vi "LV to ITX  Retrieve.vi"(0 "File or Folder Path":path, 1 "Data Type":T1=enum."TDMS", 2 "DAT header length":i32=11, 5 "offset":i32, 7 "length":i32=1, 9 "index":T2={"A"=10, "B"=6, "C"=14, "D"=1, "E"=2, "N1"=3, "N2"=2, "N3"=0, "N4"=0}, 11 "error in (no error)":errorcluster) -> (4 "A vs B":cluster{dbl[], dbl[]}[](graph), 6 "C vs D":cluster{dbl[], dbl[]}[](graph), 8 "E":dbl[][](graph), 10 "N":cluster{"N1":dbl, "N2":dbl, "N3":dbl, "N4":dbl}={"N1"=0.0624995231628418, "N2"=0.0624995231628418, "N3"=0.0624995231628418, "N4"=0.0624995231628418} {"N4" format="%#_6p"; "N3" format="%#_6p"; "N2" format="%#_6p"; "N1" format="%#_6p"}, 14 "Comments":string)   [LabVIEW 2020, in "LVtoITX.lvclass"]
uses:
  <userlib>/LevyLab/LV to ITX/LVtoITX.lvclass
  <userlib>/LevyLab/LV-Data/LV-Data.ITX/LV-Data.ITX.lvclass
  <userlib>/LevyLab/LV-Data/LV-Data.TDMS/LV-Data.TDMS.lvclass
  <userlib>/LevyLab/Graph Utilities/graph_utilities.lvclass
  <vilib>/Utility/miscctls.llb/LVOffsetAndMultiplierTypeDef.ctl
  <userlib>/LevyLab/LV-Data/LV-Data.ITX/Typedefs/Retrieve Data Type.ctl
panel:
  in  "D  is time?":bool
  in  "B is time?":bool
  out "time":string[][](table)
  in  "Use Folder Index File?":bool
  in  "Generate Folder Index File?":bool
  in  "Ez name":string="Ez name"
  in  "Ey name":string="Ey name"
  in  "Ex name":string="Ex name"
  in  "C y name":string="C y name"
  in  "D x name":string="D x name"
  in  "A y name":string="A y name"
  in  "B x name":string="B x name"
  out "Index, Wavenames":string[][](table)=[["0", "Time"], ["1", "Vsg"], ["2", "X1"], ["3", "Y1"], ["4", "X2"], ["5", "Y2"], ["6", "X3"], ["7", "Y3"], ["8", "X4"], ["9", "Y4"], ["10", "X5"], ["11", "Y5"], ["12", "X6"], ["13", "Y6"], ["14", "X7"], ["15", "Y7"], ["16", "X8"], ["17", "Y8"]]
  in  "recolor traces?":bool
  in  "Ex":T3={"Offset"=0.0, "Multiplier"=1.0}
  in  "Ey":T3={"Offset"=0.0, "Multiplier"=1.0}
  out "Path":path=path "G:/My Drive/ansom/Data/PPMSDAQ/2020/PPMS/SA02821O.20200721/04-Bsweep-Lockin/SA02821O.20200721.000000.tdms"
  out "counter":i32
  out "pattern":string="*.dat"
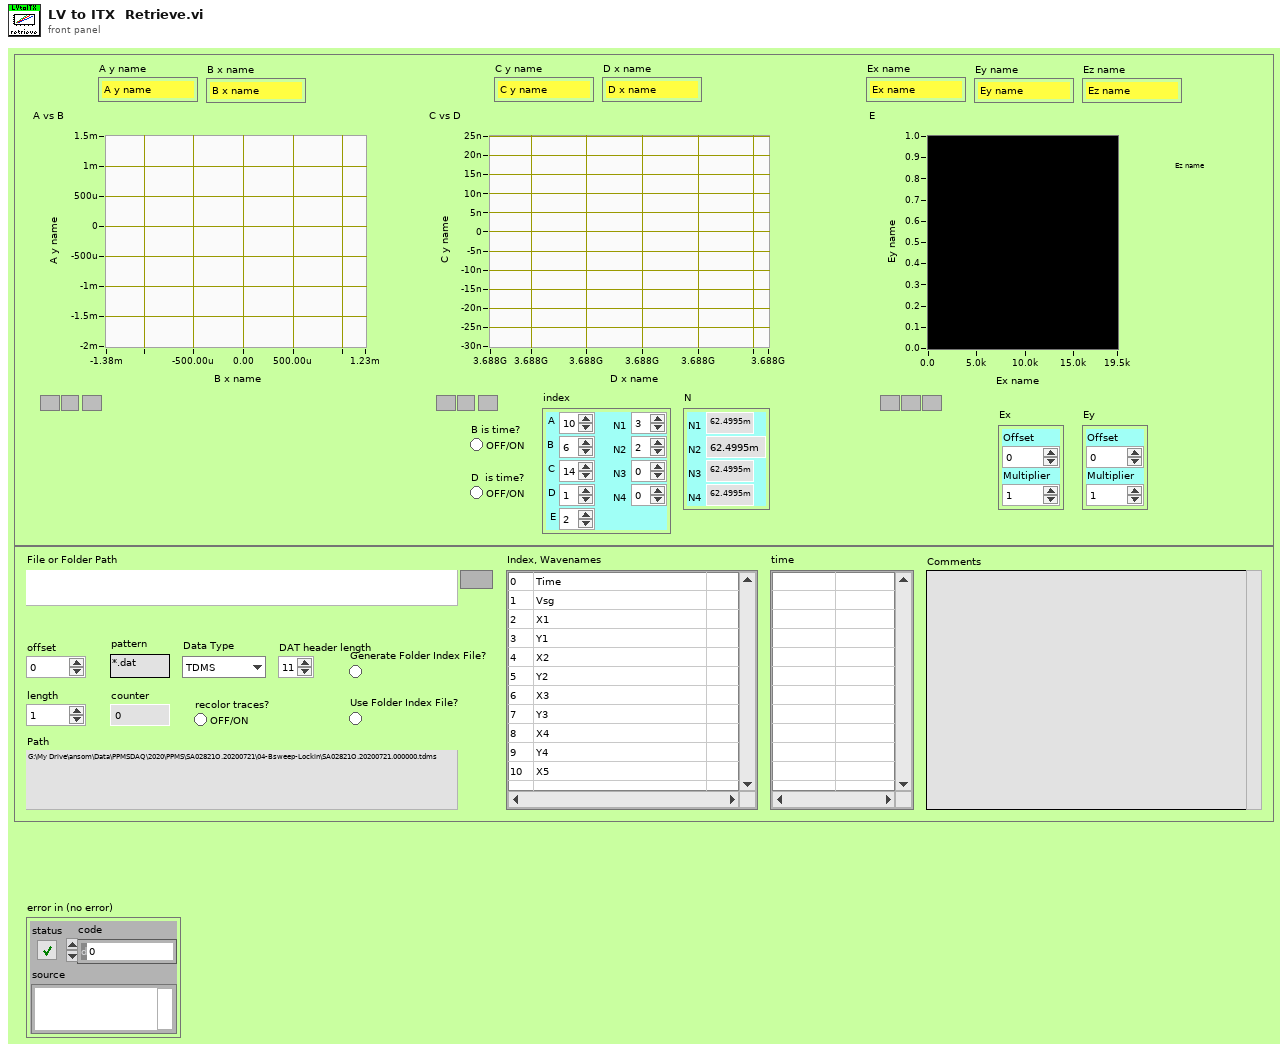
[diagram p1: front panel]
types:
  T1 = typedef "LV-Data.ITX.lvclass/Retrieve Data Type.ctl" = enum16{"ITX", "ITX w/ 2D", "DAT", "TDMS"}
  T2 = cluster{"A":i32, "B":i32, "C":i32, "D":i32, "E":i32, "N1":i32, "N2":i32, "N3":i32, "N4":i32}
  T3 = typedef "LVOffsetAndMultiplierTypeDef.ctl" = cluster{"Offset":dbl, "Multiplier":dbl}
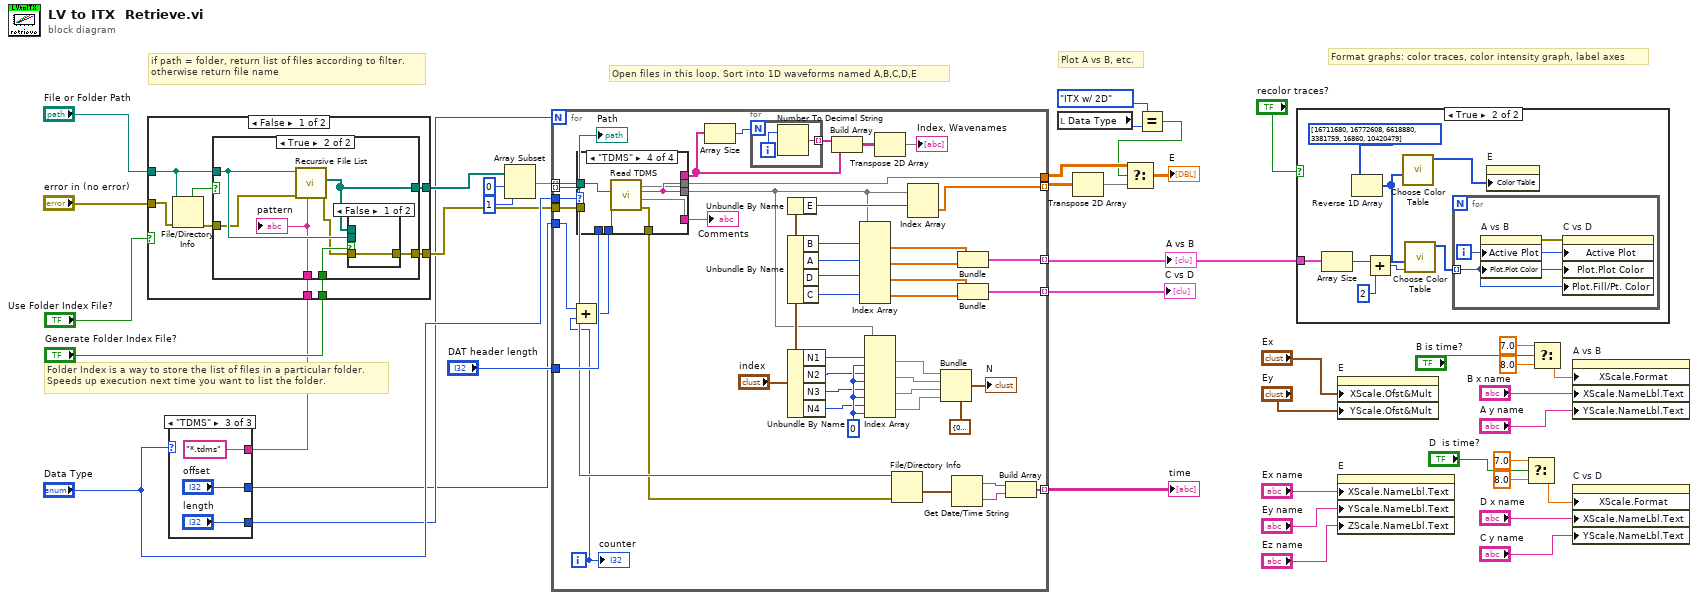
[diagram p0: block diagram]
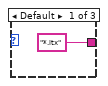
[diagram p2: hidden frame]
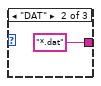
[diagram p3: hidden frame]
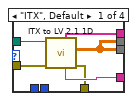
[diagram p5: hidden frame]
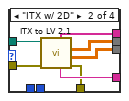
[diagram p6: hidden frame]
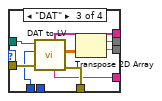
[diagram p7: hidden frame]
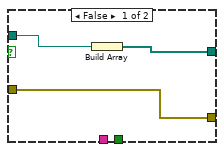
[diagram p8: hidden frame]
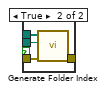
[diagram p9: hidden frame]
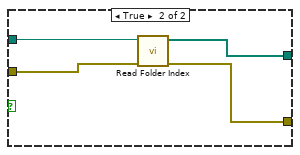
[diagram p10: hidden frame]
diagram:
  # "Plot A vs B, etc."
  # "Format graphs: color traces, color intensity graph, label axes"
  # "Open files in this loop. Sort into 1D waveforms named A,B,C,D,E"
  # "Folder Index is a way to store the list of files in a particular folder.\nSpeeds up execution next time you want to list the folder."
  # "if path = folder, return list of files according to filter.\notherwise return file name"
  n1 = case shown="\"TDMS\"" "Data Type" {
    tunnel: ["*.itx" ("pattern") "*.dat" ("pattern") "*.tdms" ("pattern")] -> w8
    tunnel: [_ _ "length"] -> w2
    tunnel: [_ _ "offset"] -> w1
    frame Default {
    }
    frame "DAT" {
    }
    frame "TDMS" {
    }
  }
  n2 = case shown="False" "Use Folder Index File?" {
    tunnel: [w53 w73] -> w40
    tunnel: "File or Folder Path" -> [w55 w74]
    tunnel: "Generate Folder Index File?" -> [w52 _]
    tunnel: w8 -> [w51 _]
    tunnel: "error in (no error)" -> [w50 w72]
    tunnel: [w48 w71] -> w5
    frame False {
      n3 = File/Directory Info(path=w55, error in=w50) -> (directory=w54:bool, error out=w49:errorcluster)  [unwired: 5 out]
      n4 = case shown="True" w54 {
        tunnel: [w58 w64] -> w53
        tunnel: w55 -> [w57 w65]
        tunnel: w52 -> [_ w61]
        tunnel: w51 -> [_ w63]
        tunnel: w49 -> [w56 w62]
        tunnel: [w56 w59] -> w48
        frame False {
          n5 = Build Array(w57) -> (w58:path[])
        }
        frame True {
          n6 = call <vilib>:"Recursive File List.vi"("pattern"=w63, "error in (no error)"=w62, "Folder Path"=w65) -> ("error out"=w60:errorcluster, "All Files in Dir"=w64:path[])  [unwired: 4 in, 3 out]
          n7 = case shown="False" w61 {
            tunnel: w64 -> [_ w70]
            tunnel: w65 -> [_ w69]
            tunnel: w60 -> [w66 w68]
            tunnel: [w66 w67] -> w59
            frame False {
            }
            frame True {
              n8 = call <userlib>:"Generate Folder Index.vi"("error in (no error)"=w68, "File or Folder Path"=w69, "All Files in Dir"=w70) -> ("error out"=w67:errorcluster)  [unwired: 8 in]
            }
          }
          "pattern" <- w63
        }
      }
    }
    frame True {
      n9 = call <userlib>:"Read Folder Index.vi"("error in (no error)"=w72, "File or Folder Path"=w74) -> ("error out"=w71:errorcluster, "Files"=w73:path[])  [unwired: 8 in]
    }
  }
  n10 = Array Subset(array=w40, index=0, length=1) -> (w21:path[])
  n11 = for {
    N: w2 -> [_]
    tunnel: w21 -> [w83] mode=indexing
    tunnel: [w83] -> _ mode=indexing
    tunnel: [w117] -> w31 mode=indexing
    tunnel: [w116] -> w30 mode=indexing
    tunnel: [w95] -> w35 mode=indexing
    tunnel: [w109] -> w33
    tunnel: [w87] -> w22 mode=indexing
    tunnel: "Data Type" -> [w85]
    tunnel: "DAT header length" -> [w84]
    tunnel: w5 -> [w82]
    tunnel: w1 -> [w76]
    i -> [w77]
    w108 = 0 ("disabled index (col)")
    n12 = Add(x=w76, y=w77) -> (x+y=w75:i32)
    n13 = case shown="\"TDMS\"" w85 {
      tunnel: [w125 w132 w134 w143] -> w118
      tunnel: [w122 w129 w140 w146] -> w88
      tunnel: w83 -> [w126 w133 w141 w147]
      tunnel: [w121 w127 w135 w145] -> w110
      tunnel: [w122 w128 w140 w146] -> w109
      tunnel: w84 -> [_ _ w136 _]
      tunnel: w82 -> [w124 w130 w139 _]
      tunnel: [w123 w131 w138 w144] -> w81
      tunnel: w75 -> [_ _ _ w142]
      frame "ITX", Default {
        n14 = call <userlib>:"ITX to LV 2.1 1D.vi"("error in"=w124, "file (use dialog)"=w126) -> ("error out"=w123:errorcluster, "1D arrays"=w122:dbl[][], "Notes"=w125:string, "base wavenames"=w121:string[])  [unwired: 4 in, 2 out]
      }
      frame "ITX w/ 2D" {
        n15 = call <userlib>:"ITX to LV 2.1.vi"("error in"=w130, "file (use dialog)"=w133) -> ("error out"=w131:errorcluster, "1D arrays"=w129:dbl[][], "2D array"=w128:dbl[][], "Notes"=w132:string, "wave names"=w127:string[])  [unwired: 3 in, 2 out]
      }
      frame "DAT" {
        n16 = call <userlib>:"DAT to LV.vi"("error in (no error)"=w139, "header length"=w136, "File Path"=w141) -> ("error out"=w138:errorcluster, "Data"=w137:dbl[][], "Comments"=w134:string, "Wavenames"=w135:string[])  [unwired: 4 in, 1 out]
        n17 = Transpose 2D Array(2D array=w137) -> (transposed array=w140:dbl[][])
      }
      frame "TDMS" {
        n18 = call <userlib>:"Read TDMS.vi"(9:w142, 10:w147) -> ("error out"=w144:errorcluster, "Notes"=w146:string, 4:w143, 5:w145)  [unwired: 4 in, 2 out]
      }
    }
    "Comments" <- w118
    n19 = Array Size(array=w110) -> (size(s)=w78:i32)
    n20 = for {
      N: w78 -> [_]
      tunnel: [w119] -> w114 mode=indexing
      i -> [w120]
      n21 = Number To Decimal String(number=w120) -> (decimal integer string=w119:string)  [unwired: 1 in]
    }
    n22 = Unbundle By Name("index") -> ("E"=w100:i32)
    n23 = Unbundle By Name("index") -> ("B"=w99:i32, "A"=w98:i32, "D"=w97:i32, "C"=w96:i32)
    n24 = Unbundle By Name("index") -> ("N1"=w101:i32, "N2"=w102:i32, "N3"=w103:i32, "N4"=w104:i32)
    n25 = Build Array(w114, w110) -> (w111:string[][])
    n26 = Index Array(array=w88, index (row) #1=w99, index (row) #2=w98, index (row) #3=w97, index (row) #4=w96) -> (element #1=w93:dbl[], element #2=w92:dbl[], element #3=w112:dbl[], element #4=w115:dbl[])  [unwired: 4 in]
    n27 = Index Array(array=w88, index (row) #1=w101, index (col) #1=w108, index (row) #2=w102, index (col) #2=w108, index (row) #3=w103, index (col) #3=w108, index (row) #4=w104, index (col) #4=w108) -> (element #1=w89:dbl, element #2=w90:dbl, element #3=w91:dbl, element #4=w107:dbl)
    n28 = Transpose 2D Array(2D array=w111) -> (transposed array=→"Index, Wavenames":string[][])
    n29 = File/Directory Info(path=w83, error in=w81) -> (last mod=w86:timestamp)  [unwired: 6 out]
    n30 = Index Array(array=w88, index (row)=w100) -> (element=w95:dbl[])  [unwired: 1 in]
    n31 = Bundle(cluster=cluster{"N1":dbl, "N2":dbl, "N3":dbl, "N4":dbl} {"N1"=0.0, "N2"=0.0, "N3"=0.0, "N4"=0.0}, "N1"=w89, "N2"=w90, "N3"=w91, "N4"=w107) -> (→"N":cluster{"N1":dbl, "N2":dbl, "N3":dbl, "N4":dbl})
    n32 = Get Date/Time String(seconds (now)=w86) -> (date string=w79:string, time string=w80:string)  [unwired: 2 in]
    n33 = Bundle("1D arrays"=w93, "1D arrays"=w92) -> (w117:cluster{"1D arrays":dbl[], "1D arrays":dbl[]})  [unwired: 1 in]
    n34 = Bundle("1D arrays"=w112, "1D arrays"=w115) -> (w116:cluster{"1D arrays":dbl[], "1D arrays":dbl[]})  [unwired: 1 in]
    n35 = Build Array(w79, w80) -> (w87:string[])
    "counter" <- w77
    "Path" <- w83
  }
  "A vs B" <- w31
  "C vs D" <- w30
  "time" <- w22
  n36 = local read "Data Type"() -> (w11:T1)
  n37 = Transpose 2D Array(2D array=w35) -> (transposed array=w36:dbl[][])
  n38 = Equal?(x=enum16{"ITX", "ITX w/ 2D", "DAT"}."ITX w/ 2D" ("Enum"), y=w11) -> (x = y?=w9:bool)
  n39 = Select(t=w33, s=w9, f=w36) -> (s? t:f=→"E":dbl[][])
  n40 = case shown="True" "recolor traces?" {
    tunnel: w31 -> [_ w150]
    frame False {
    }
    frame True {
      n41 = Array Size(array=w150) -> (size(s)=w151:i32)
      n42 = Reverse 1D Array(array=u32[] [16711680, 16772608, 6618880, 3381759, 16860, 10420479] ("color scale")) -> (reversed array=w149:u32[])
      n43 = Add(x=w151, y=2 ("x")) -> (x+y=w155:i32)
      n44 = call <userlib>:"Choose Color Table.vi"("Custom Table"=w149) -> ("Color Table"=w153:u32[])  [unwired: 7 in, 3 out]
      n45 = call <userlib>:"Choose Color Table.vi"("Size (256)"=w155, "Custom Table"=w149) -> ("Color Table"=w152:u32[])  [unwired: 6 in, 3 out]
      n46 = for {
        tunnel: w152 -> [w156] mode=indexing
        i -> [w157]
        n47 = property on="A vs B" class="XYGraph (strict)"("Active Plot"=w157, "Plot.Plot Color"=w156) -> (error out=w158:errorcluster)  [unwired: 2 in, 1 out]
        n48 = property on="C vs D" class="XYGraph (strict)"(error in=w158, "Active Plot"=w157, "Plot.Plot Color"=w156, "Plot.Fill/Pt. Color"=w156) -> ()  [unwired: 1 in, 2 out]
      }
      n49 = property on="E" class="IntGraph (strict)"("Color Table"=w153) -> ()  [unwired: 2 in, 2 out]
    }
  }
  n50 = property on="E" class="IntGraph (strict)"("XScale.Ofst&Mult"="Ex", "YScale.Ofst&Mult"="Ey") -> ()  [unwired: 2 in, 2 out]
  n51 = property on="E" class="IntGraph (strict)"("XScale.NameLbl.Text"="Ex name", "YScale.NameLbl.Text"="Ey name", "ZScale.NameLbl.Text"="Ez name") -> ()  [unwired: 2 in, 2 out]
  n52 = Select(t=7.0, s="D  is time?", f=8.0) -> (s? t:f=w17:dbl)
  n53 = Select(t=7.0, s="B is time?", f=8.0) -> (s? t:f=w18:dbl)
  n54 = property on="A vs B" class="XYGraph (strict)"("XScale.Format"=w18, "XScale.NameLbl.Text"="B x name", "YScale.NameLbl.Text"="A y name") -> ()  [unwired: 2 in, 2 out]
  n55 = property on="C vs D" class="XYGraph (strict)"("XScale.Format"=w17, "XScale.NameLbl.Text"="D x name", "YScale.NameLbl.Text"="C y name") -> ()  [unwired: 2 in, 2 out]
